vi "SwerveModuleState_New.vi"(9 "ROTATION":T1={"VALUE"=0.0, "COS"=1.0, "SIN"=0.0} {"SIN" format="%13.4f"; "COS" format="%13.4f"; "VALUE" format="%13.4f"}, 11 "Speed":dbl) -> (3 "SWERVE_DRIVE_MODULE_STATE":T2={"Speed"=0.0, "Angle"={"VALUE"=0.0, "COS"=1.0, "SIN"=0.0}} {"Angle"."SIN" format="%13.4f"; "Angle"."COS" format="%13.4f"; "Angle"."VALUE" format="%13.4f"})   [LabVIEW 2019, in "Trajectory_Library.lvlib"]
doc: "Constructs a SwerveModuleState.\n \nParameters:\n - speed - The speed of the wheel of the module. (Meters/Sec)\n - rotation -The angle of the module.\n\nReturns:\n - SwerveDriveModuleState - Data structure"
uses:
  Trajectory_Library.lvlib
  TypeDef/ROTATION2D.ctl
  TypeDef/SWERVE_DRIVE_MODULE_STATE.ctl
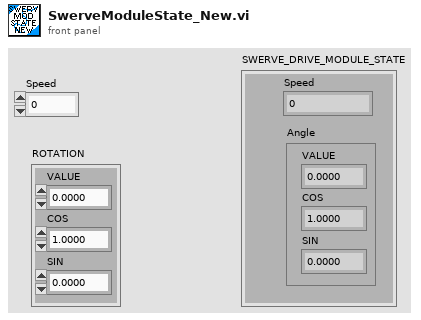
[diagram p1: front panel]
types:
  T1 = typedef "Trajectory_Library.lvlib/ROTATION2D.ctl" = cluster{"VALUE":dbl, "COS":dbl, "SIN":dbl}
  T2 = typedef "Trajectory_Library.lvlib/SWERVE_DRIVE_MODULE_STATE.ctl" = cluster{"Speed":dbl, "Angle":T1}
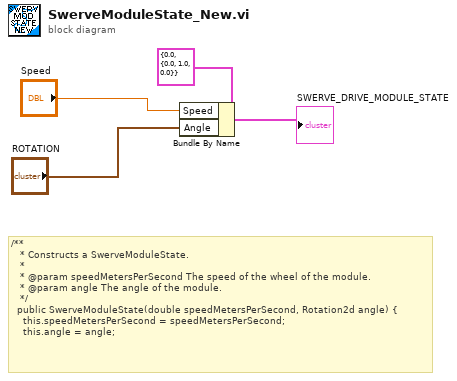
[diagram p0: block diagram]
diagram:
  # "/**\n   * Constructs a SwerveModuleState.\n   *\n   * @param speedMetersPerSecond The speed of the wheel of the module.\n   * @param angle The angle of the module.\n   */\n  public SwerveModuleState(double speedMetersPerSecond, Rotation2d angle) {\n    this.speedMetersPerSecond = speedMetersPerSecond;\n    this.angle = angle;"
  n1 = Bundle By Name(cluster=T2 {"Speed"=0.0, "Angle"={"VALUE"=0.0, "COS"=1.0, "SIN"=0.0}} ("SWERVE_DRIVE_MODULE_STATE"), "Speed"="Speed", "Angle"="ROTATION") -> (→"SWERVE_DRIVE_MODULE_STATE":T2)
